vi "Get System Time.vi"(8 "error in (no error)":errorcluster, 11 "Embedded Data Logger System Tests in":refnum<class "Embedded Data Logger System Tests.lvclass">) -> (0 "error out":errorcluster, 2 "System Time":dbl, 3 "Embedded Data Logger System Tests out":refnum<class "Embedded Data Logger System Tests.lvclass">)   [LabVIEW 2018, in "Embedded Data Logger System Tests.lvclass"]
uses:
  Embedded Data Logger System Tests.lvclass
  C:/Dev/niveristand-custom-device-testing-tools/VeriStandTestCase/VeriStandTestCase.lvclass
  <vilib>/NI Veristand/Execution/Workspace/NI VeriStand - Get Single Channel Value.vi
  <vilib>/NI Veristand/Execution/Workspace/NI_VS Workspace ExecutionAPI.lvlib
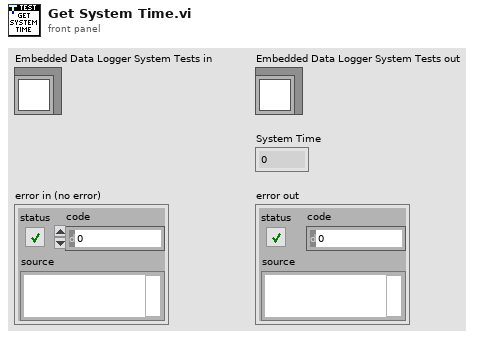
[diagram p1: front panel]
types:
  T1 = typedef "NI_VS Workspace ExecutionAPI.lvlib/WorkspaceAPI.ctl" = refnum<k24>
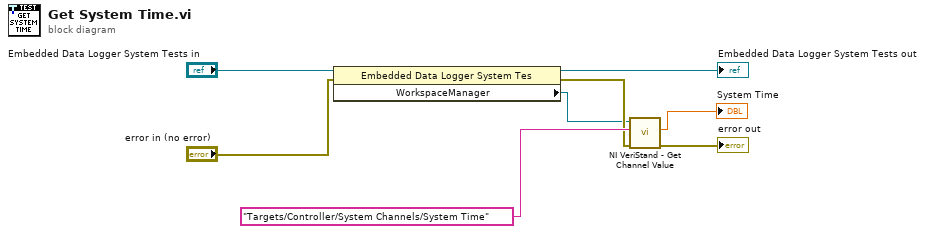
[diagram p0: block diagram]
diagram:
  n1 = property class="Embedded Data Logger System Tes"(reference="Embedded Data Logger System Tests in", error in="error in (no error)") -> (reference out=→"Embedded Data Logger System Tests out":refnum<class "Embedded Data Logger System Tests.lvclass">, error out=w5:errorcluster, "WorkspaceManager"=w4:T1)
  n2 = call-poly <vilib>:"NI VeriStand - Get Channel Value.vi"("error in (no error)"=w5, "Channel"="Targets/Controller/System Channels/System Time", "WorkspaceManager in"=w4) -> ("error out"=→"error out":errorcluster, "Value"=→"System Time":dbl)  [unwired: 6 in, 1 out]
